vi "Equi-Ripple BandPass PtByPt.vi"(0 "x":dbl format="%0.2f", 1 "lower pass freq":dbl=0.25000000000000006 format="%0.2f", 2 "higher pass freq":dbl=0.3500000000000001 format="%0.2f", 3 "initialize":bool, 7 "sampling freq: fs":dbl=1.0 format="%0.2f", 11 "# of taps":i32=32, 12 "lower stop freq":dbl=0.2 format="%0.2f", 13 "higher stop freq":dbl=0.4000000000000001 format="%0.2f") -> (4 "Filtered x":dbl format="%0.2f", 15 "error":i32)   [LabVIEW 2020, in "NI_PtbyPt.lvlib"]
doc: "Filters <B>x</B> using an equi-ripple bandpass FIR filter model."
uses:
  NI_PtbyPt.lvlib
  NI_AALBase.lvlib
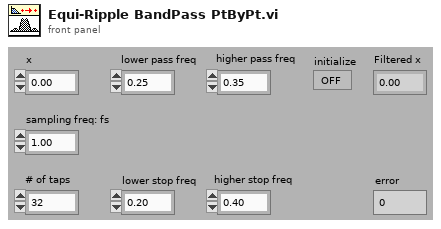
[diagram p1: front panel]
types:
  T1 = cluster{"Amplitude":dbl, "DC":dbl, "lower stop freq":dbl, "Weight":dbl}
  T2 = cluster{"Amplitude":dbl, "lower pass freq":dbl, "higher pass freq":dbl, "Weight":dbl}
  T3 = cluster{"Amplitude":dbl, "higher stop freq":dbl, dbl, "Weight":dbl}
  T4 = cluster{"Amplitude":dbl, "higher stop freq":dbl, "higher pass freq":dbl, "Weight":dbl}[]
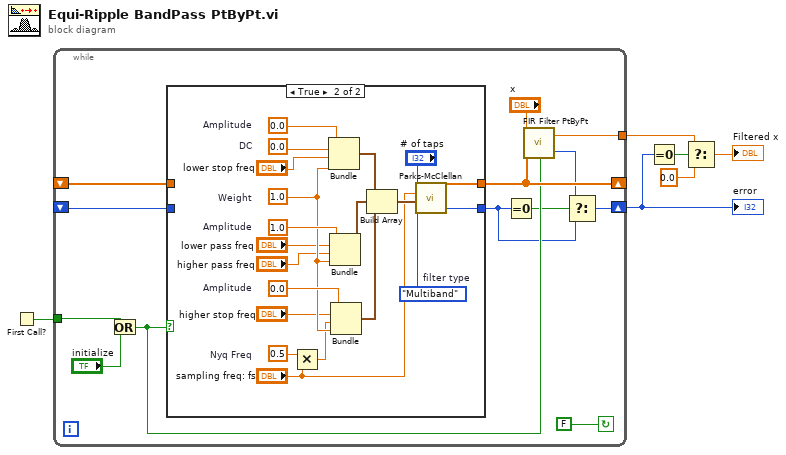
[diagram p0: block diagram]
diagram:
  n1 = First Call?() -> (First Call?: T/F=w6:bool)
  n2 = while {
    tunnel: w6 -> [w15]
    shift-left: _ -> [w17]
    shift-right: [w19] -> _
    shift-right: [w9] -> w5
    shift-left: _ -> [w8]
    tunnel: [w7] -> w3
    stop <- FALSE continue-if-true
    n3 = Or(x=w15, y="initialize") -> (x .or. y?=w13:bool)
    n4 = case shown="True" w13 {
      tunnel: [w21 w41] -> w19
      tunnel: w17 -> [w21 _]
      tunnel: [w20 w22] -> w10
      tunnel: w8 -> [w20 _]
      frame False {
      }
      frame True {
        w35 = 0.0  # Amplitude
        w36 = 0.0  # DC
        w37 = 1.0  # Weight
        w38 = 1.0  # Amplitude
        w40 = 0.5  # Nyq Freq
        w39 = 0.0  # Amplitude
        w34 = enum32{"Multiband", "Differentiator", "Hilbert"}."Multiband"  # filter type
        n5 = Multiply(x=w40, y="sampling freq: fs") -> (x*y=w30:dbl)
        n6 = Bundle("Amplitude"=w35, "DC"=w36, "lower stop freq"="lower stop freq", "Weight"=w37) -> (w25:T1)  [unwired: 1 out]
        n7 = Bundle("Amplitude"=w38, "lower pass freq"="lower pass freq", "higher pass freq"="higher pass freq", "Weight"=w37) -> (w26:T2)  [unwired: 1 out]
        n8 = Bundle("Amplitude"=w39, "higher stop freq"="higher stop freq", w30, "Weight"=w37) -> (w31:T3)  [unwired: 1 out]
        n9 = Build Array(w25, w26, w31) -> (w33:T4)
        n10 = call "Parks-McClellan.vi"("filter type"=w34, "Band Parameters"=w33, "sampling freq: fs"="sampling freq: fs", "# of taps"="# of taps") -> ("error"=w22:i32, "h"=w41:dbl[])  [unwired: 1 out]
      }
    }
    n11 = Equal To 0?(x=w10) -> (x = 0?=w12:bool)
    n12 = call "FIR Filter PtByPt.vi"("initialize"=w13, "Forward Coefficients"=w19, "x"="x") -> ("error"=w11:i32, "Filtered x"=w7:dbl)  [unwired: 1 out]
    n13 = Select(t=w11, s=w12, f=w10) -> (s? t:f=w9:i32)
  }
  "error" <- w5
  n14 = Equal To 0?(x=w5) -> (x = 0?=w4:bool)
  n15 = Select(t=w3, s=w4, f=0.0) -> (s? t:f=→"Filtered x":dbl)
